vi "StahlPS_Pbus.SetVoltage.vi"(0 "i ref in":refnum<vi>, 2 "value":dbl, 5 "error in (no error)":errorcluster, 7 "channelIndex":i32) -> (14 "i ref out":refnum<vi>, 19 "error out (no error)":errorcluster)   [LabVIEW 2014, in "StahlPS_Pbus.lvlib"]
doc: "This VI calculates the right current from the DB values, saves the actual set current to the I-Attribute and set´s the Set Current-Service."
uses:
  StahlPS_Pbus.lvlib
  CSCore/CSSystem/CoreDefs/CoreDefs.error_type.ctl
  CSCore/CSSystem/CoreDefs/CoreDefs.error_severity.ctl
  CSCore/CSApplicationBaseClasses/PSChannelBase/PSChannelBase.directionType.ctl
  CSCore/CSApplicationBaseClasses/PSChannelBase/PSChannelBase.serviceType.ctl
  CSlibraries/UtilityLib/UtilityLib.valueStatus.ctl
  CSCore/CSSystem/CoreLib/CoreLib.lvlib
  CSlibraries/UtilityLib/UtilityLib.lvlib
  CSCore/CSApplicationBaseClasses/PSChannelBase/PSChannelBase.lvlib
  CSlibraries-extern/DimLVEvent/LVDimInterface/LVDimInterface.lvlib
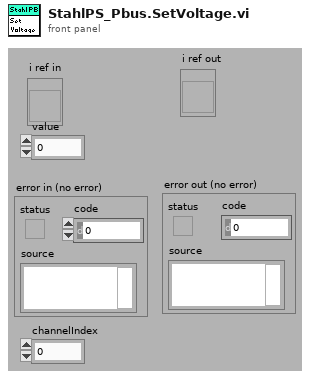
[diagram p1: front panel]
types:
  T1 = typedef "CoreDefs.error_severity.ctl" = enum16{"undefined", "information", "warning", "error", "fatal"}
  T2 = typedef "CoreDefs.error_type.ctl" = enum16{"no error", "can't load process", "can't unload process", "process does not exist", "can't install process", "can't remove process", "unknown function", "time out", "can't execute function", "duplicate queue name", "super not found", "caller queue invalid", "can't ping process", "unknown error", "VISA Error", "VISA timeout", "GPIB timeout", "GPIB error", "communication error", "data type mismatch", "can't read data from OPC server", "can't write data to OPC server", "OET error", "function not implemented", "process already exists", "invalid Shared Variable name", "error writing Shared Variable", "error reading Shared Variable", "invalid client name", "corrupt database", "unknown class", "call not authorized", "parameter out of range", "OET timeout: can't get data to modify", "invalid queue name", "requested operation incompatible with current state", "event undefined", "event disabled", "state undefined", "caller is not a friend", "EventBuilder: bad eventID", "EventBuilder: no DAQ devices", "a thread must not stop itself", "UNUSED ELEMENT4", "DiscArchiver: eventData incomplete", "DiscArchiver: eventData does not belong to run", "DiscArchiver: can't open file", "DiscArchiver: can't write to file", "DiscArchiver: available disc space low", "can't acquire semaphore", "error reading data from database", "notifier object is not existing", "can't register process", "can't unregister process", "illegal event type", "object disabled", "object already exists", "can't change state", "Instrument not found", "no connection to remote node", "invalid reference", "N/A", "UNUSED ELEMENT 1", "element not found", "illegal TCP/IP connection detected", "object does not exist", "invalid access ID", "unknown CS system", "invalid privilige", "unsupported data type", "unsupported server type", "IO server already exists", "Shared Variable already exists"}
  T3 = typedef "UtilityLib.lvlib/UtilityLib.valueStatus.ctl" = enum16{"no info available", "stand by/off", "on", "warning", "alarm/malfunction", "not implemented", "user action required", "important information", "system default", "control default", "indicator default", "button default"}
  T4 = typedef "PSChannelBase.lvlib/PSChannelBase.serviceType.ctl" = enum16{"onOff", "voltage", "current", "tripCurrent", "rampUpSpeed", "rampDownSpeed", "status"}
  T5 = typedef "PSChannelBase.lvlib/PSChannelBase.directionType.ctl" = enum16{"unknown", "update actual value", "update nominal value", "update both"}
  T6 = typedef "StahlPS_Pbus.lvlib/StahlPS_Pbus.i attribute.ctl" = cluster{"Type":string, "CALC_FACTOR_SET_VOLTAGE":dbl, "CALC_FACTOR_GET_VOLTAGE":dbl, "CALC_FACTOR_GET_CURRENT":dbl, "CALC_FACTOR_SET_CURRENT ":dbl, "REG_VALUE":dbl, "Sign":bool, "setVoltIDs":i32[], "Elektrode Names":string[]}
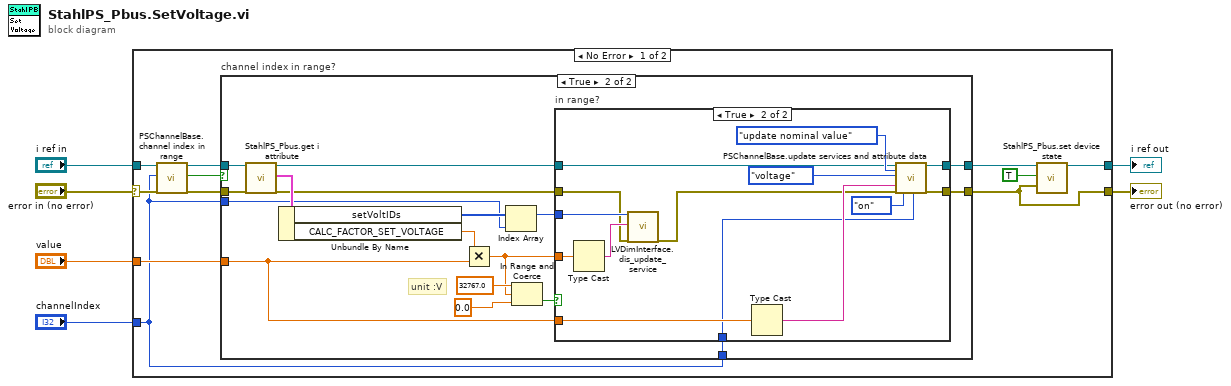
[diagram p0: block diagram]
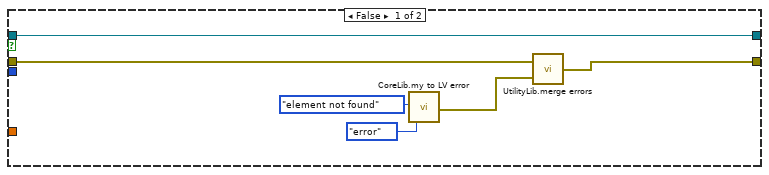
[diagram p2: hidden frame]
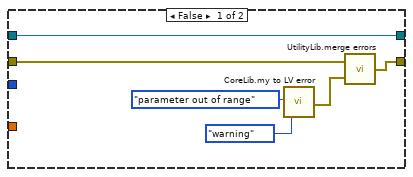
[diagram p3: hidden frame]
diagram:
  n1 = case shown="No Error" "error in (no error)" {
    selector: "error in (no error)" -> [w16 w62]
    tunnel: [w10 w62] -> w3
    tunnel: "i ref in" -> [w15 w61]
    tunnel: [w9 w61] -> w5
    tunnel: "value" -> [w17 _]
    tunnel: "channelIndex" -> [w7 _]
    frame No Error {
      n2 = call "PSChannelBase.channel index in range.vi"("i ref in"=w15, "channelIndex"=w7, "error in (no error)"=w16) -> ("i ref out"=w12:refnum<vi>, "in range"=w13:bool, "error out"=w14:errorcluster)  [unwired: 14 in]
      n3 = case "channel index in range?" shown="True" w13 {
        tunnel: w12 -> [w23 w34]
        tunnel: [w23 w33] -> w11
        tunnel: w14 -> [w20 w32]
        tunnel: [w18 w31] -> w10
        tunnel: w17 -> [_ w27]
        tunnel: w7 -> [_ w26]
        tunnel: w7 -> [_ w24]
        frame False {
          n4 = call "CoreLib.my to LV error.vi"("ErrorTypes"=CoreDefs.error_type."element not found", "severityLevel"=CoreDefs.error_severity."error") -> ("myErrorCluster"=w19:errorcluster)  [unwired: 16 in, 1 out]
          n5 = call "UtilityLib.merge errors.vi"("error2 (no error)"=w19, "error1 (no error)"=w20) -> ("error out"=w18:errorcluster)
        }
        frame True {
          # "unit :V"
          n6 = call "StahlPS_Pbus.get i attribute.vi"("i ref in"=w34, "error in (no error)"=w32) -> ("i ref out"=w29:refnum<vi>, "i attribute"=w40:T6, "error out"=w30:errorcluster)  [unwired: 15 in]
          n7 = Unbundle By Name(w40) -> ("setVoltIDs"=w28:i32[], "CALC_FACTOR_SET_VOLTAGE"=w39:dbl)
          n8 = Multiply(x=w39, y=w27) -> (x*y=w35:dbl)
          n9 = Index Array(array=w28, index=w24) -> (element=w25:i32)
          n10 = In Range and Coerce(upper limit=32767.0, x=w35, lower limit=0.0 ("upper limit")) -> (In Range?=w38:bool)  [unwired: 1 out]
          n11 = case "in range?" shown="True" w38 {
            tunnel: w30 -> [w44 w52]
            tunnel: [w42 w59] -> w31
            tunnel: w35 -> [_ w47]
            tunnel: w29 -> [w41 w50]
            tunnel: [w41 w60] -> w33
            tunnel: w25 -> [_ w54]
            tunnel: w27 -> [_ w51]
            tunnel: w26 -> [_ w48]
            frame False {
              n12 = call "CoreLib.my to LV error.vi"("ErrorTypes"=CoreDefs.error_type."parameter out of range", "severityLevel"=CoreDefs.error_severity."warning") -> ("myErrorCluster"=w43:errorcluster)  [unwired: 16 in, 1 out]
              n13 = call "UtilityLib.merge errors.vi"("error2 (no error)"=w43, "error1 (no error)"=w44) -> ("error out"=w42:errorcluster)
            }
            frame True {
              n14 = Type Cast(x=w47) -> (*(type *) &x=w53:string)  [unwired: 1 in]
              n15 = call "LVDimInterface.dis_update_service.vi"("my_serviceID"=w54, "data"=w53, "error in (no error)"=w52) -> ("error out"=w49:errorcluster)  [unwired: 14 in, 2 out]
              n16 = Type Cast(x=w51) -> (*(type *) &x=w58:string)  [unwired: 1 in]
              n17 = call "PSChannelBase.update services and attribute data.vi"("i ref in"=w50, "direction"=PSChannelBase.directionType."update nominal value", "service"=PSChannelBase.serviceType."voltage", "value"=w58, "error in (no error)"=w49, "quality"=UtilityLib.valueStatus."on", "channelNumber"=w48) -> ("i ref out"=w60:refnum<vi>, "error out"=w59:errorcluster)  [unwired: 10 in, 1 out]
            }
          }
        }
      }
      n18 = call "StahlPS_Pbus.set device state.vi"("i ref in"=w11, "implicit"=TRUE, "device error"=w10) -> ("i ref out"=w9:refnum<vi>)  [unwired: 14 in, 2 out]
    }
    frame Error {
    }
  }
  "error out (no error)" <- w3
  "i ref out" <- w5
